vi "TDC_configureSelftest.vi"(0 "Channel Mask":i32, 5 "Period [5ns]":i32=2 min=2 max=60, 7 "Burst Size":i32=1 min=1 max=65535, 9 "Burst Distance [20 ns]":i32 min=0 max=10000, 11 "Error In":errorcluster) -> (15 "Error Out":errorcluster)   [LabVIEW 2011]
uses:
  tdcbase.dll
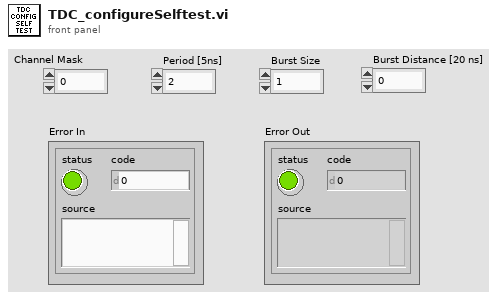
[diagram p1: front panel]
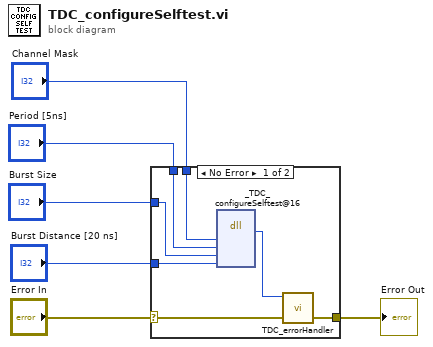
[diagram p0: block diagram]
diagram:
  n1 = case shown="No Error" "Error In" {
    selector: "Error In" -> [w9 w14]
    tunnel: [w8 w14] -> w5
    tunnel: "Channel Mask" -> [w13 _]
    tunnel: "Period [5ns]" -> [w12 _]
    tunnel: "Burst Size" -> [w11 _]
    tunnel: "Burst Distance [20 ns]" -> [w10 _]
    frame No Error {
      n2 = dll-call lib="X:/tdcbase.dll" fn="_TDC_configureSelftest@16"("channelMask"=w13, "period"=w12, "burstSize"=w11, "burstDist"=w10) -> ("return type"=w7:i32)  [unwired: 7 in, 2 out]
      n3 = call "TDC_errorHandler.vi"("Error In"=w9, "TDC Return Code"=w7) -> ("Error Out"=w8:errorcluster)  [unwired: 9 in]
    }
    frame Error {
    }
  }
  "Error Out" <- w5
